vi "Automatic Teller Machine (ATM).vi"() -> ()   [LabVIEW 2018]
panel:
  in  "输入":bool
  in  "用户输入":string
  in  "右按钮":cluster{"功能按钮":bool, "功能按钮2":bool, "功能按钮3":bool}
  out "右菜单":T1
  in  "左按钮":cluster{"功能按钮":bool, "功能按钮2":bool, "功能按钮3":bool}
  out "左菜单":T1
  in  "卡模拟器":bool
  out "ATM消息":string
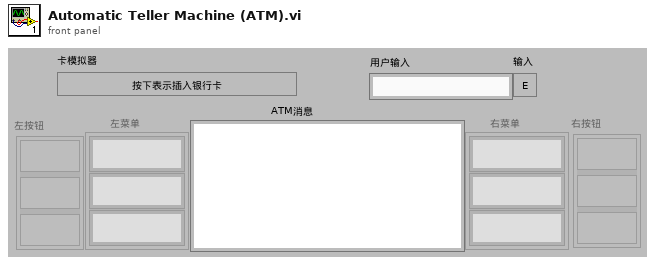
[diagram p1: front panel]
types:
  T1 = cluster{"RFS字符串":string, "RFS字符串2":string, "RFS字符串3":string}
  T2 = typedef "输入状态.ctl" = enum16{"输入密码", "输入取款金额", "输入存款金额"}
  T3 = typedef "账户信息.ctl" = cluster{"密码":string, "名字":string, "姓氏":string, "余额":dbl}
  T4 = typedef "状态.ctl" = enum16{"初始化", "等待"}
  T5 = enum8{"Enabled", "Disabled", "Disabled and Grayed Out"}
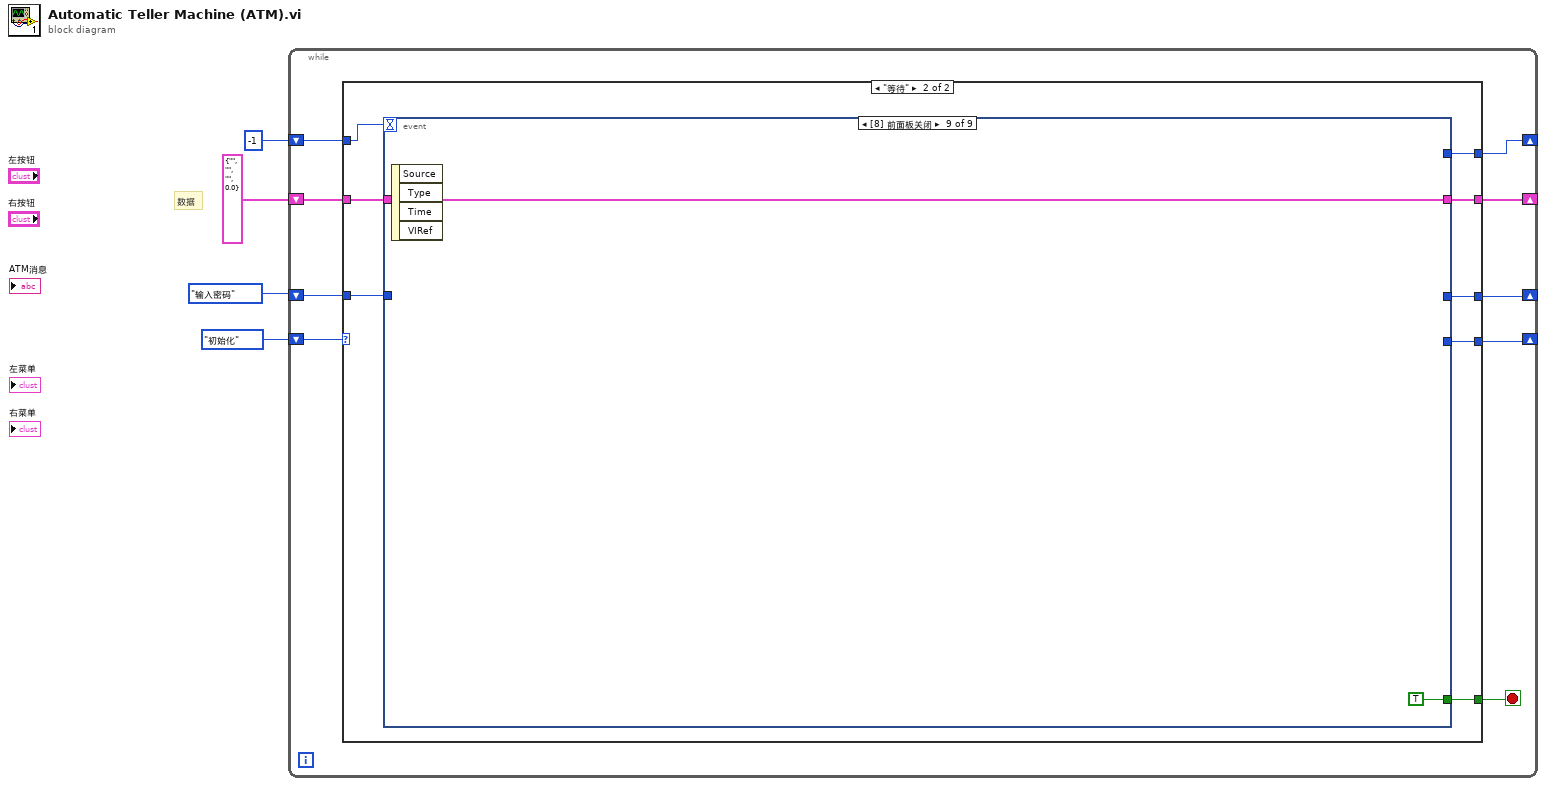
[diagram p0: block diagram]
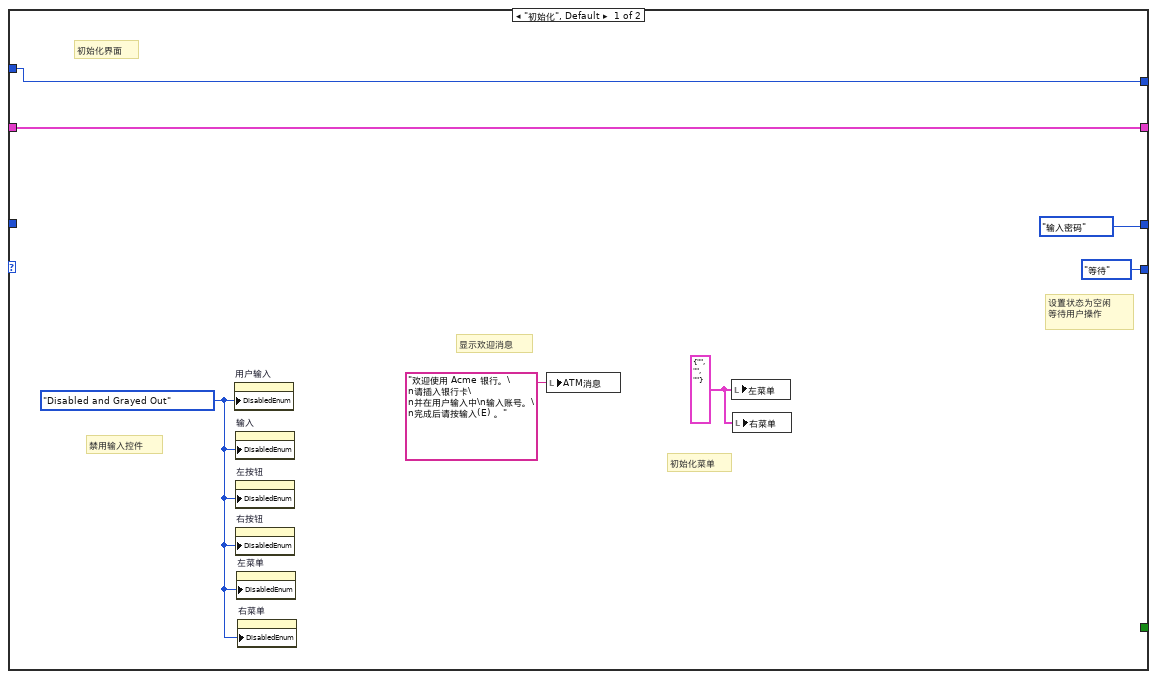
[diagram p2: hidden frame]
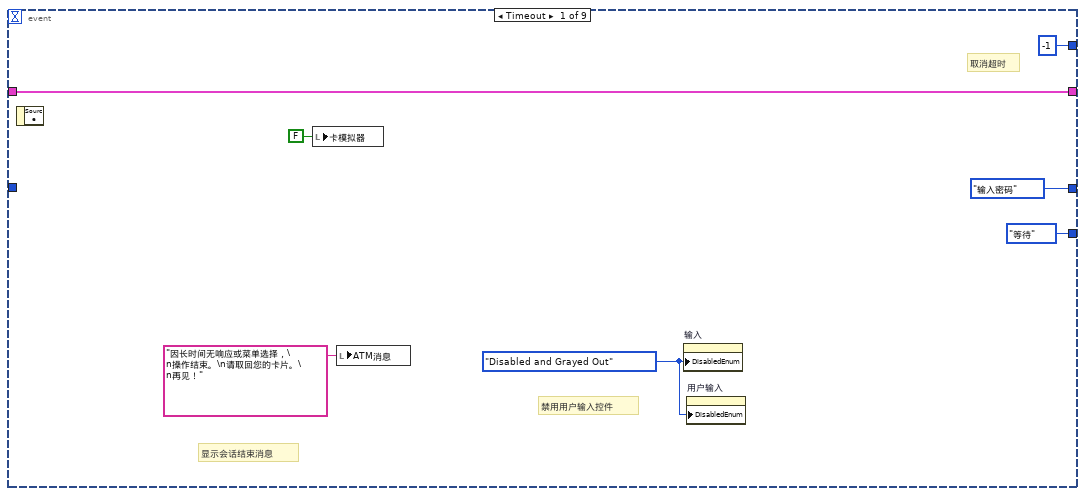
[diagram p3: hidden frame]
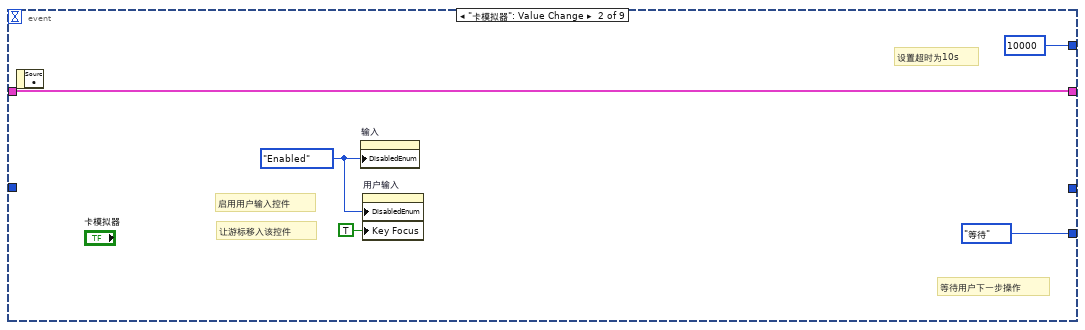
[diagram p4: hidden frame]
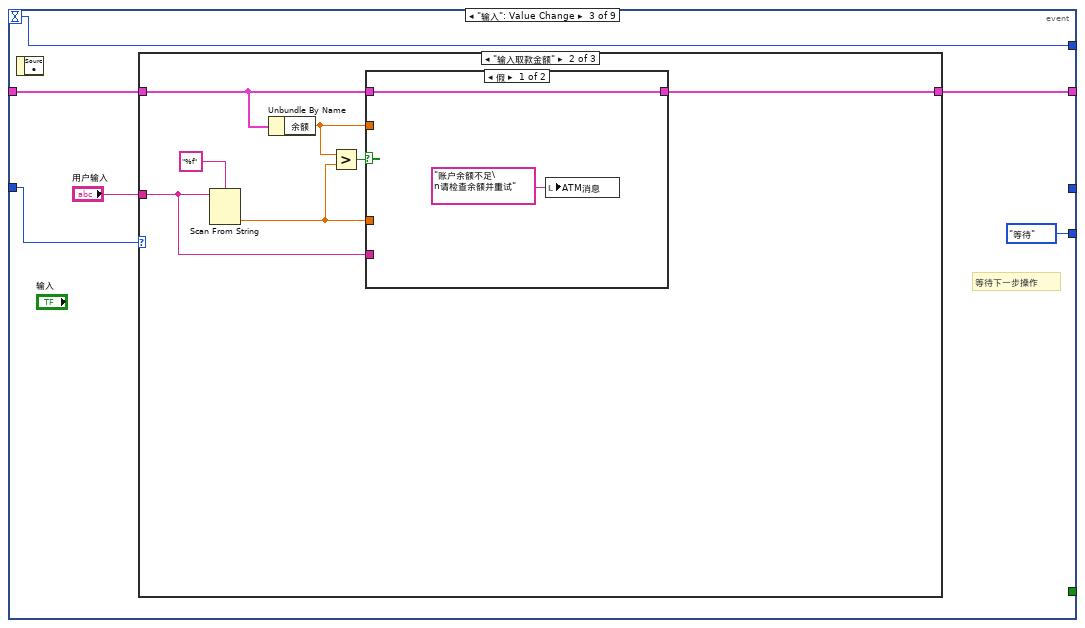
[diagram p5: hidden frame]
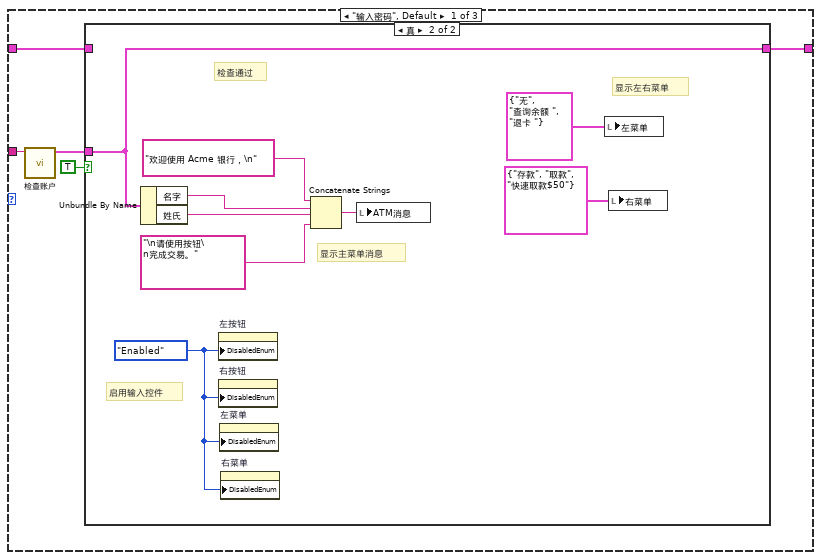
[diagram p6: hidden frame]
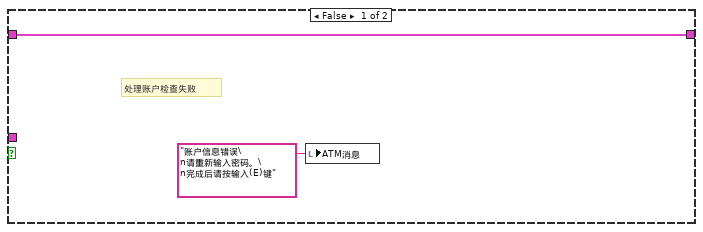
[diagram p7: hidden frame]
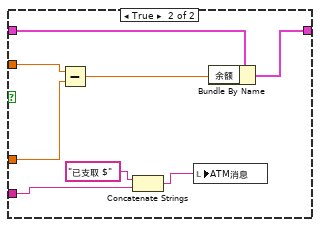
[diagram p8: hidden frame]
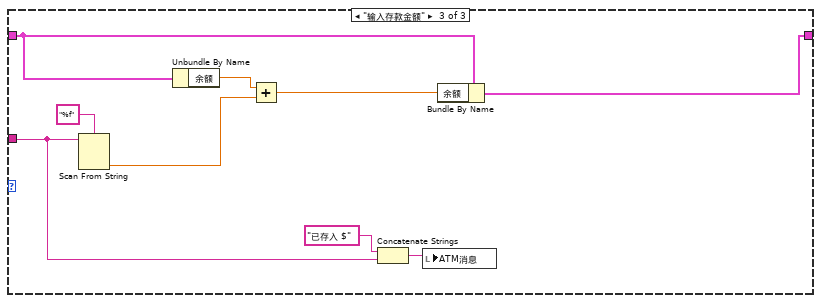
[diagram p9: hidden frame]
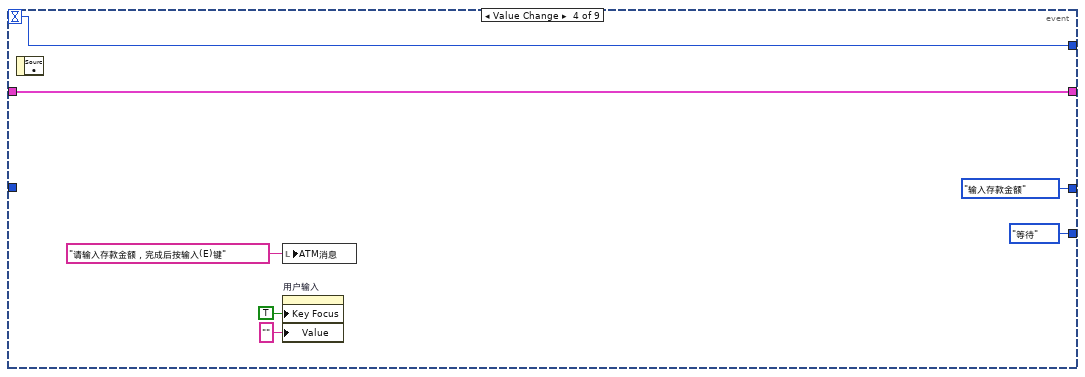
[diagram p10: hidden frame]
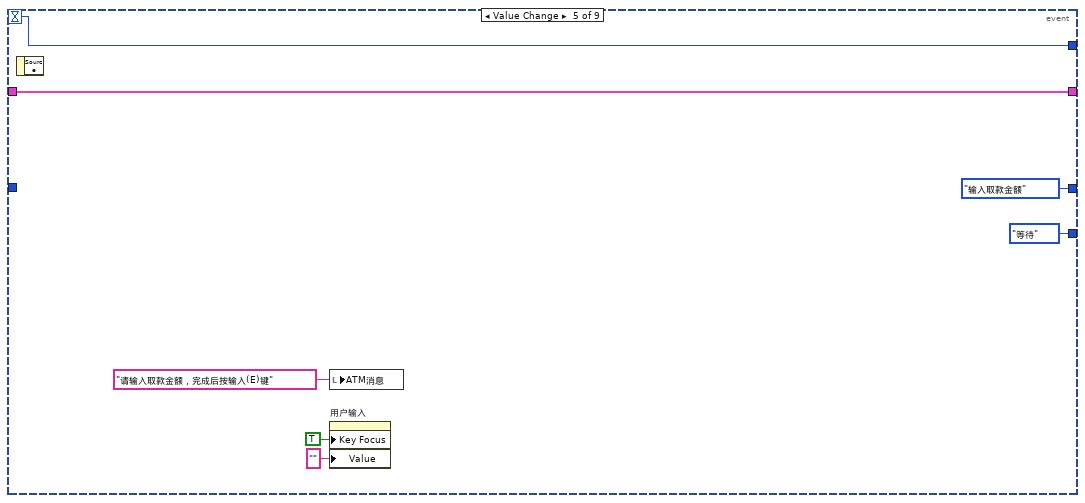
[diagram p11: hidden frame]
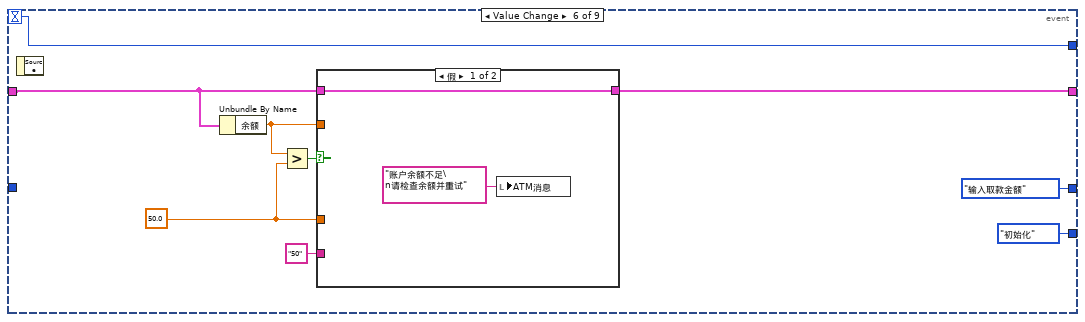
[diagram p12: hidden frame]
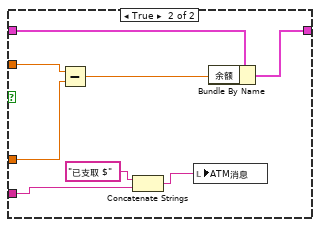
[diagram p13: hidden frame]
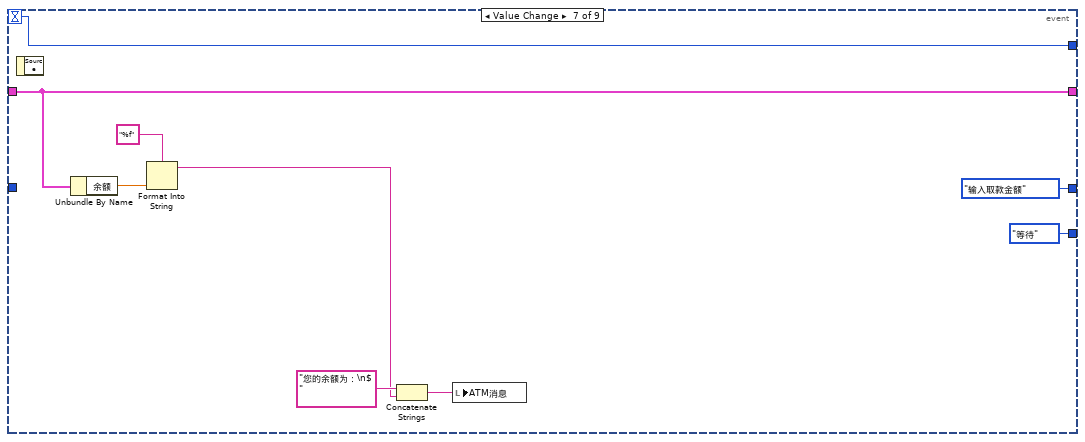
[diagram p14: hidden frame]
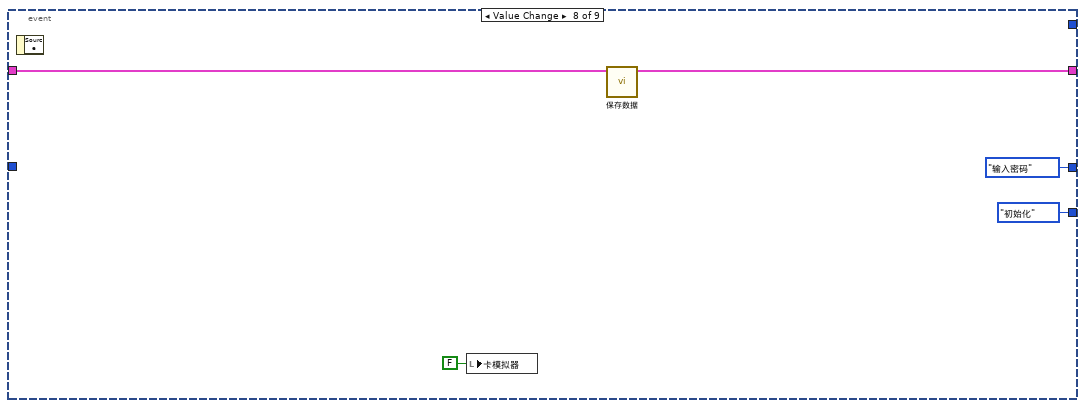
[diagram p15: hidden frame]
diagram:
  # "数据"
  n1 = while {
    shift-right: [w12] -> _
    shift-left: 状态."初始化" ("状态") -> [w13]
    shift-right: [w9] -> _
    shift-left: -1 -> [w10]
    shift-right: [w8] -> _
    shift-left: T3 {"密码"="", "名字"="", "姓氏"="", "余额"=0.0} ("账户信息") -> [w7]
    shift-right: [w5] -> _
    shift-left: 输入状态."输入密码" ("状态") -> [w6]
    stop <- w11 stop-if-true
    n2 = case shown="\"等待\"" w13 {
      tunnel: [状态."等待" ("状态") w28] -> w12
      tunnel: [_ w21] -> w11
      tunnel: w10 -> [w16 w27]
      tunnel: [w16 w26] -> w9
      tunnel: [w15 w25] -> w8
      tunnel: w7 -> [w15 w24]
      tunnel: w6 -> [_ w23]
      tunnel: [输入状态."输入密码" ("状态") w22] -> w5
      frame "初始化", Default {
        w17 = T1 {"RFS字符串"="", "RFS字符串2"="", "RFS字符串3"=""} ("左菜单")
        w19 = T5."Disabled and Grayed Out" ("禁用")
        # "初始化菜单"
        # "显示欢迎消息"
        # "设置状态为空闲\n等待用户操作"
        # "禁用输入控件"
        # "初始化界面"
        n3 = property on="用户输入" class="Str"("DisabledEnum"=w19) -> ()  [unwired: 2 in, 2 out]
        n4 = property on="输入" class="Bool"("DisabledEnum"=w19) -> ()  [unwired: 2 in, 2 out]
        n5 = property on="左按钮" class="Clust"("DisabledEnum"=w19) -> ()  [unwired: 2 in, 2 out]
        n6 = property on="右按钮" class="Clust"("DisabledEnum"=w19) -> ()  [unwired: 2 in, 2 out]
        n7 = property on="左菜单" class="Clust (严格)"("DisabledEnum"=w19) -> ()  [unwired: 2 in, 2 out]
        n8 = property on="右菜单" class="Clust (严格)"("DisabledEnum"=w19) -> ()  [unwired: 2 in, 2 out]
        n9 = local write "ATM消息"("欢迎使用 Acme 银行。\n请插入银行卡\n并在用户输入中\n输入账号。\n完成后请按输入(E) 。" ("ATM消息")) -> ()
        n10 = local write "左菜单"(w17) -> ()
        n11 = local write "右菜单"(w17) -> ()
      }
      frame "等待" {
        n12 = event shown="[8] 前面板关闭" {
          selector: _ -> [_ _ _ _ _ _ _ _ _]
          dyn-events: _ -> [_ _ _ _ _ _ _ _ _]
          timeout: w27 -> [_ _ w46 w94 w96 w103 w129 _ _]
          tunnel: [状态."等待" ("状态") 状态."等待" ("状态") 状态."等待" ("状态") 状态."等待" ("状态") 状态."等待" ("状态") 状态."初始化" ("状态") 状态."等待" ("状态") 状态."初始化" ("状态") _] -> w28
          tunnel: [-1 10000 w46 w94 w96 w103 w129 _ _] -> w26
          tunnel: [w30 w36 w44 w95 w102 w104 w127 w131 w137] -> w25
          tunnel: w24 -> [w30 w36 w45 w95 w102 w107 w127 w132 w137]
          tunnel: w23 -> [_ _ w41 _ _ _ _ _ _]
          tunnel: [输入状态."输入密码" ("状态") _ _ 输入状态."输入存款金额" ("状态") 输入状态."输入取款金额" ("状态") 输入状态."输入取款金额" ("状态") 输入状态."输入取款金额" ("状态") 输入状态."输入密码" ("状态") _] -> w22
          tunnel: [_ _ _ _ _ _ _ _ TRUE] -> w21
          event Timeout {
            w32 = T5."Disabled and Grayed Out" ("禁用")
            # "显示会话结束消息"
            # "禁用用户输入控件"
            # "取消超时"
            n13 = event-data() -> ()  [unwired: 1 in, 1 out]
            n14 = local write "卡模拟器"(FALSE ("卡模拟器")) -> ()
            n15 = local write "ATM消息"("因长时间无响应或菜单选择，\n操作结束。\n请取回您的卡片。\n再见！" ("ATM消息")) -> ()
            n16 = property on="输入" class="Bool"("DisabledEnum"=w32) -> ()  [unwired: 2 in, 2 out]
            n17 = property on="用户输入" class="Str"("DisabledEnum"=w32) -> ()  [unwired: 2 in, 2 out]
          }
          event "卡模拟器": Value Change {
            w39 = T5."Enabled" ("禁用")
            # "等待用户下一步操作"
            # "设置超时为10s"
            # "让游标移入该控件"
            # "启用用户输入控件"
            n18 = event-data() -> ()  [unwired: 1 in, 1 out]
            n19 = property on="输入" class="Bool"("DisabledEnum"=w39) -> ()  [unwired: 2 in, 2 out]
            n20 = property on="用户输入" class="Str"("DisabledEnum"=w39, "Key Focus"=TRUE ("键选中")) -> ()  [unwired: 2 in, 2 out]
          }
          event "输入": Value Change {
            # "等待下一步操作"
            n21 = event-data() -> ()  [unwired: 1 in, 1 out]
            n22 = case shown="\"输入取款金额\"" w41 {
              tunnel: w45 -> [w51 w67 w87]
              tunnel: [w50 w66 w86] -> w44
              tunnel: "用户输入" -> [w49 w65 w80]
              frame "输入密码", Default {
                n23 = call "检查账户.vi"("密码"=w49) -> ("账户信息"=w48:T3)  [unwired: 9 in, 1 out]
                n24 = case shown="真" TRUE {
                  tunnel: w51 -> [w53 _]
                  tunnel: [w53 w60] -> w50
                  tunnel: w48 -> [_ w60]
                  frame False {
                    # "处理账户检查失败"
                    n25 = local write "ATM消息"("账户信息错误\n请重新输入密码。\n完成后请按输入(E)键" ("ATM消息")) -> ()
                  }
                  frame True {
                    w56 = T5."Enabled" ("禁用")
                    # "显示左右菜单"
                    # "启用输入控件"
                    # "显示主菜单消息"
                    # "检查通过"
                    n26 = Unbundle By Name(w60) -> ("名字"=w59:string, "姓氏"=w58:string)
                    n27 = property on="左按钮" class="Clust"("DisabledEnum"=w56) -> ()  [unwired: 2 in, 2 out]
                    n28 = property on="右按钮" class="Clust"("DisabledEnum"=w56) -> ()  [unwired: 2 in, 2 out]
                    n29 = property on="左菜单" class="Clust (严格)"("DisabledEnum"=w56) -> ()  [unwired: 2 in, 2 out]
                    n30 = property on="右菜单" class="Clust (严格)"("DisabledEnum"=w56) -> ()  [unwired: 2 in, 2 out]
                    n31 = Concatenate Strings("欢迎使用 Acme 银行，\n" ("ATM消息"), w59, w58, "\n请使用按钮\n完成交易。" ("ATM消息")) -> (w57:string)
                    n32 = local write "ATM消息"(w57) -> ()
                    n33 = local write "左菜单"(T1 {"RFS字符串"="无", "RFS字符串2"="查询余额 ", "RFS字符串3"="退卡 "} ("左菜单")) -> ()
                    n34 = local write "右菜单"(T1 {"RFS字符串"="存款", "RFS字符串2"="取款", "RFS字符串3"="快速取款$50"} ("右菜单")) -> ()
                  }
                }
              }
              frame "输入取款金额" {
                n35 = Scan From String(format string="%f" ("格式字符串"), input string=w65) -> (output 1=w63:dbl)  [unwired: 3 in, 3 out]
                n36 = Unbundle By Name(w67) -> ("余额"=w64:dbl)
                n37 = Greater?(x=w64, y=w63) -> (0:w68:bool)
                n38 = case shown="假" w68 {
                  tunnel: w67 -> [w71 w79]
                  tunnel: [w71 w78] -> w66
                  tunnel: w65 -> [_ w76]
                  tunnel: w64 -> [_ w74]
                  tunnel: w63 -> [_ w73]
                  frame False {
                    n39 = local write "ATM消息"("账户余额不足\n请检查余额并重试" ("ATM消息")) -> ()
                  }
                  frame True {
                    n40 = Subtract(x=w74, y=w73) -> (x-y=w72:dbl)
                    n41 = Concatenate Strings("已支取 $" ("ATM消息"), w76) -> (w75:string)
                    n42 = local write "ATM消息"(w75) -> ()
                    n43 = Bundle By Name(cluster=w79, "余额"=w72) -> (w78:T3)
                  }
                }
              }
              frame "输入存款金额" {
                n44 = Scan From String(format string="%f" ("格式字符串"), input string=w80) -> (output 1=w84:dbl)  [unwired: 3 in, 3 out]
                n45 = Unbundle By Name(w87) -> ("余额"=w85:dbl)
                n46 = Add(x=w85, y=w84) -> (x+y=w83:dbl)
                n47 = Concatenate Strings("已存入 $" ("ATM消息"), w80) -> (w81:string)
                n48 = local write "ATM消息"(w81) -> ()
                n49 = Bundle By Name(cluster=w87, "余额"=w83) -> (w86:T3)
              }
            }
          }
          event "右按钮.功能按钮": Value Change {
            n50 = event-data() -> ()  [unwired: 1 in, 1 out]
            n51 = local write "ATM消息"("请输入存款金额，完成后按输入(E)键" ("ATM消息")) -> ()
            n52 = property on="用户输入" class="Str"("Key Focus"=TRUE ("键选中"), "Value"="" ("用户输入")) -> ()  [unwired: 2 in, 2 out]
          }
          event "右按钮.功能按钮2": Value Change {
            n53 = event-data() -> ()  [unwired: 1 in, 1 out]
            n54 = local write "ATM消息"("请输入取款金额，完成后按输入(E)键" ("ATM消息")) -> ()
            n55 = property on="用户输入" class="Str"("Key Focus"=TRUE ("键选中"), "Value"="" ("用户输入")) -> ()  [unwired: 2 in, 2 out]
          }
          event "右按钮.功能按钮3": Value Change {
            w106 = 50.0 ("y")
            n56 = event-data() -> ()  [unwired: 1 in, 1 out]
            n57 = Unbundle By Name(w107) -> ("余额"=w108:dbl)
            n58 = Greater?(x=w108, y=w106) -> (0:w109:bool)
            n59 = case shown="假" w109 {
              tunnel: w107 -> [w113 w121]
              tunnel: [w113 w120] -> w104
              tunnel: "50" ("用户输入") -> [_ w118]
              tunnel: w108 -> [_ w116]
              tunnel: w106 -> [_ w115]
              frame False {
                n60 = local write "ATM消息"("账户余额不足\n请检查余额并重试" ("ATM消息")) -> ()
              }
              frame True {
                n61 = Subtract(x=w116, y=w115) -> (x-y=w114:dbl)
                n62 = Concatenate Strings("已支取 $" ("ATM消息"), w118) -> (w117:string)
                n63 = local write "ATM消息"(w117) -> ()
                n64 = Bundle By Name(cluster=w121, "余额"=w114) -> (w120:T3)
              }
            }
          }
          event "左按钮.功能按钮2": Value Change {
            n65 = event-data() -> ()  [unwired: 1 in, 1 out]
            n66 = Unbundle By Name(w127) -> ("余额"=w126:dbl)
            n67 = Format Into String(format string="%f" ("格式字符串"), w126) -> (resulting string=w123:string)  [unwired: 2 in, 1 out]
            n68 = Concatenate Strings("您的余额为：\n$ " ("ATM消息"), w123) -> (w122:string)
            n69 = local write "ATM消息"(w122) -> ()
          }
          event "左按钮.功能按钮3": Value Change {
            n70 = event-data() -> ()  [unwired: 1 in, 1 out]
            n71 = local write "卡模拟器"(FALSE ("卡模拟器")) -> ()
            n72 = call "保存数据.vi"("账户信息"=w132) -> ("账户信息 2"=w131:T3)  [unwired: 10 in]
          }
          event Panel Close {
            n73 = event-data() -> ()  [unwired: 1 in, 4 out]
          }
        }
      }
    }
  }
